vi "Change Real Point.vi"(7 "MultiList Ref":refnum<vi>, 8 "error in (no error)":errorcluster, 10 "Y":dbl, 11 "X":dbl) -> (0 "error out":errorcluster, 4 "All Real Points":cluster{dbl, dbl}[](array[cluster]))   [LabVIEW 2015]
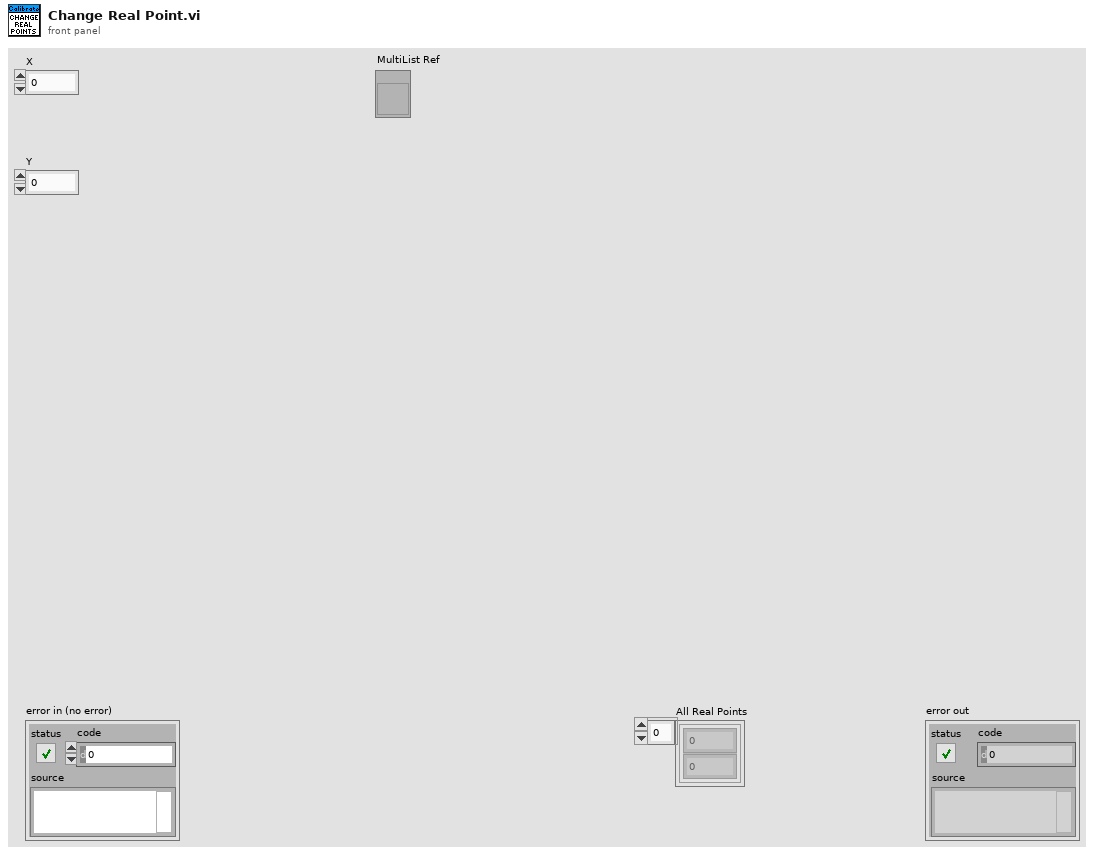
[diagram p1: front panel]
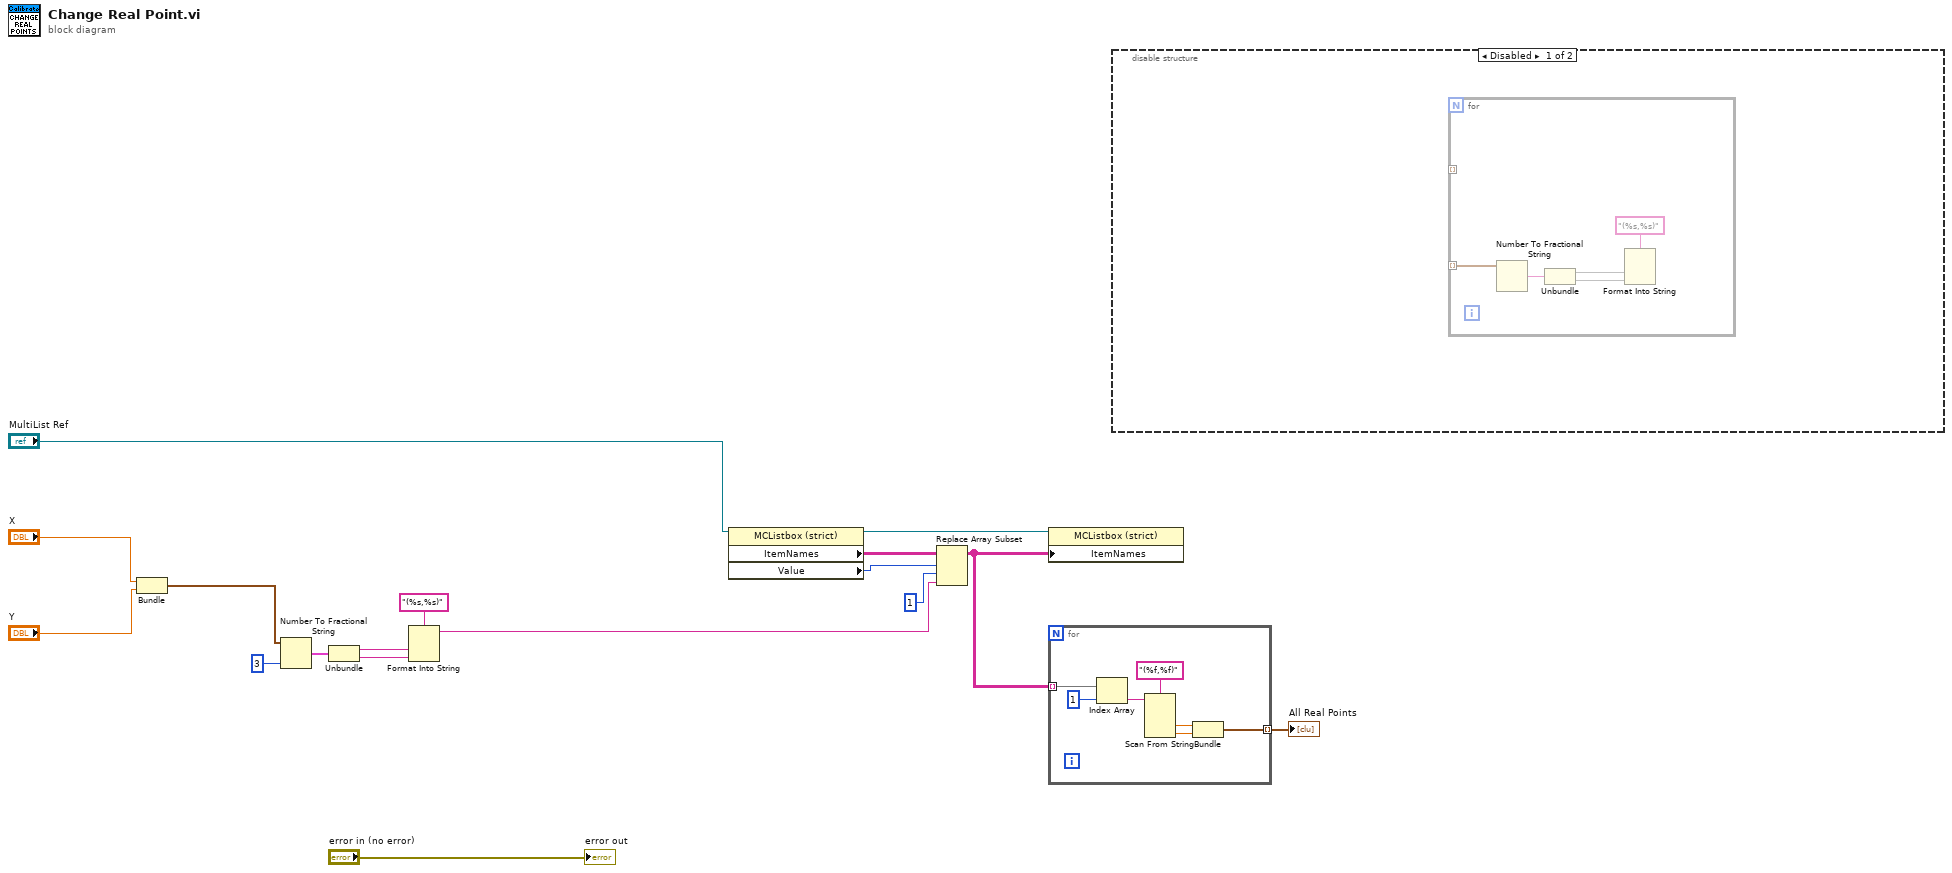
[diagram p0: block diagram]
diagram:
  n1 = Bundle("X"="X", "Y"="Y") -> (w8:cluster{"X":dbl, "Y":dbl})  [unwired: 1 in]
  n2 = Number To Fractional String(number=w8, precision (6)=i16 3) -> (F-format string=w11:cluster{"X":string, "Y":string})  [unwired: 2 in]
  n3 = Unbundle(w11) -> ("X"=w12:string, "Y"=w13:string)
  n4 = Format Into String(format string="(%s,%s)", w12, w13) -> (resulting string=w4:string)  [unwired: 2 in, 1 out]
  n5 = property class="MCListbox (strict)"(reference="MultiList Ref") -> (reference out=w3:refnum<vi>, "ItemNames"=w6:string[][], "Value"=w7:i32)  [unwired: 1 in, 1 out]
  n6 = Replace Array Subset(array=w6, new element=w4, index (row)=w7, index (col)=1 ("disabled index (col)")) -> (w2:string[][])
  n7 = property class="MCListbox (strict)"(reference=w3, "ItemNames"=w2) -> ()  [unwired: 1 in, 2 out]
  n8 = for {
    tunnel: w2 -> [w22] mode=indexing
    tunnel: [w19] -> w1 mode=indexing
    n9 = Index Array(array=w22, index=1) -> (element=w24:string)
    n10 = Scan From String(format string="(%f,%f)", input string=w24) -> (output 1=w20:dbl, output 2=w21:dbl)  [unwired: 4 in, 3 out]
    n11 = Bundle(w20, w21) -> (w19:cluster{dbl, dbl})  [unwired: 1 in]
  }
  "All Real Points" <- w1
  n12 = disable-structure shown="Disabled" {
    frame Disabled {
      n13 = for {
        tunnel: [_] -> w25 mode=indexing
        tunnel: [w33] -> w26 mode=indexing
        n14 = Number To Fractional String(number=w33) -> (precision (6)=w27:i16, F-format string=w29:string)  [unwired: 2 in]
        n15 = Unbundle(w29) -> (w30, w31)
        n16 = Format Into String(format string="(%s,%s)", w30, w31) -> (resulting string=w28:string)  [unwired: 2 in, 1 out]
      }
    }
    frame Enabled {
    }
  }
  "error out" <- "error in (no error)"
